vi "test Port Setup.vi"(8 "error in (no error)":errorcluster, 11 "TestCase in":refnum<class "AIM ARINC 664 Port Setup.lvclass">) -> (0 "error out":errorcluster, 3 "TestCase out":refnum<class "AIM ARINC 664 Port Setup.lvclass">)   [LabVIEW 2020, in "AIM ARINC 664 Port Setup.lvclass"]
uses:
  AIM ARINC 664 Port Setup.lvclass
  C:/Program Files (x86)/National Instruments/LabVIEW 2020/vi.lib/addons/_JKI Toolkits/VI Tester/TestCase.llb/TestCase.lvclass
  AIM ARINC 664 Port Setup.lvclass/AIM ARINC 664 Port Setup.ctl
  <vilib>/addons/_JKI Toolkits/VI Tester/TestCase.llb/TestCase.lvclass
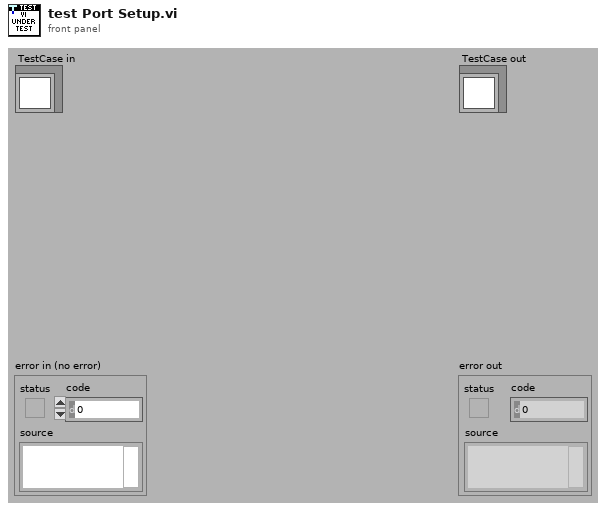
[diagram p1: front panel]
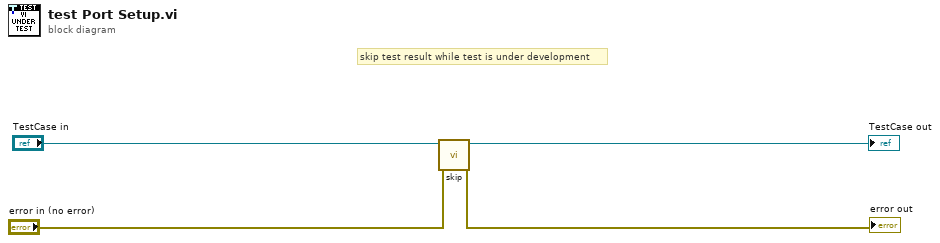
[diagram p0: block diagram]
diagram:
  # "skip test result while test is under development"
  n1 = call <vilib>:"skip.vi"("error in (no error)"="error in (no error)", "TestCase in"="TestCase in") -> ("error out"=→"error out":errorcluster, "TestCase out"=→"TestCase out":refnum<class "AIM ARINC 664 Port Setup.lvclass">)  [unwired: 8 in]
